vi "Project Save As.vi"(8 "error in (no error)":errorcluster, 9 "Rename Items[]":T1[](array[typedef]), 10 "Existing Project Path":path, 11 "New Project Path":path) -> (0 "error out":errorcluster)   [LabVIEW 2016, in "SLL Scripting.lvlib"]
uses:
  SLL Scripting.lvlib
  _Typedefs/Rename Item Cluster.ctl
  <vilib>/Utility/EditLVProj/Edit LVProj.lvlib
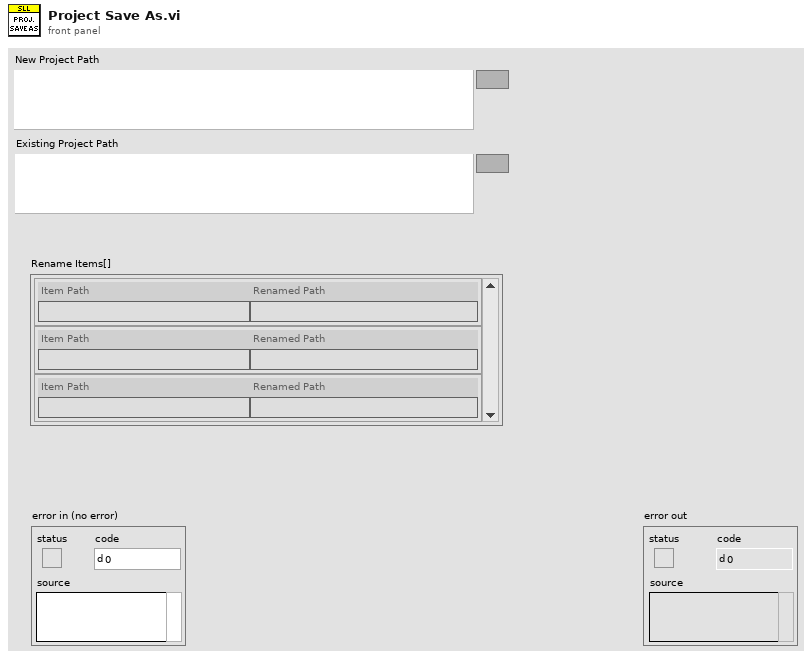
[diagram p1: front panel]
types:
  T1 = typedef "Rename Item Cluster.ctl" = cluster{"Item Path":string, "Renamed Path":string}
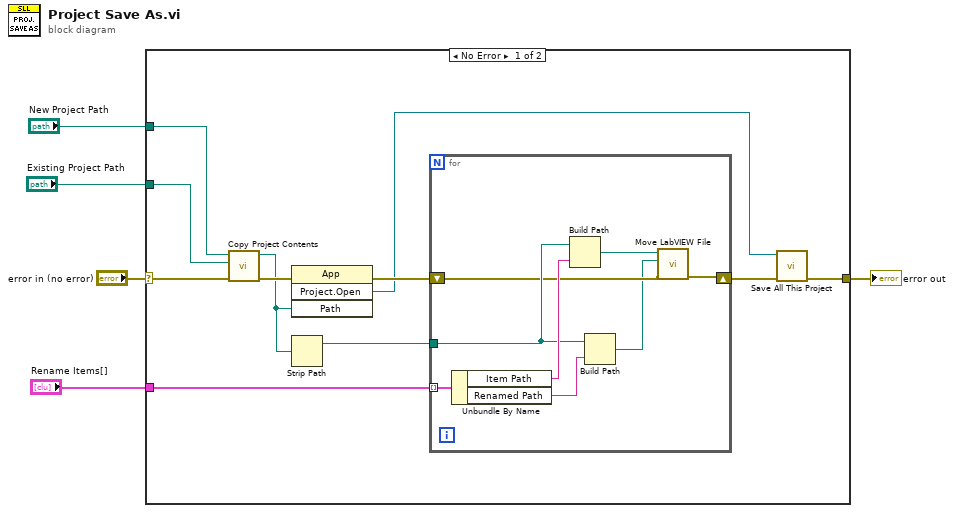
[diagram p0: block diagram]
diagram:
  n1 = case shown="No Error" "error in (no error)" {
    selector: "error in (no error)" -> [w16 w25]
    tunnel: [w7 w25] -> w4
    tunnel: "Existing Project Path" -> [w14 _]
    tunnel: "New Project Path" -> [w15 _]
    tunnel: "Rename Items[]" -> [w11 _]
    frame No Error {
      n2 = call "Copy Project Contents.vi"("error in (no error)"=w16, "Existing Project Path"=w14, "New Project Path"=w15) -> ("error out"=w13:errorcluster, "New Project Path Out"=w10:path)  [unwired: 7 in]
      n3 = invoke class="App" method="Project.Open"(error in=w13, "Path"=w10) -> (error out=w12:errorcluster, "Project:Open"=w6:refnum<vi>)  [unwired: 2 in, 2 out]
      n4 = Strip Path(path=w10) -> (stripped path=w9:path)  [unwired: 1 out]
      n5 = for {
        shift-right: [w17] -> w8
        shift-left: w12 -> [w20]
        tunnel: w11 -> [w24] mode=indexing
        tunnel: w9 -> [w22]
        n6 = Unbundle By Name(w24) -> ("Item Path"=w23:string, "Renamed Path"=w21:string)
        n7 = Build Path(base path=w22, name or relative path=w23) -> (appended path=w19:path)
        n8 = Build Path(base path=w22, name or relative path=w21) -> (appended path=w18:path)
        n9 = call "Move LabVIEW File.vi"("error in (no error)"=w20, "New Path"=w18, "Existing Path"=w19) -> ("error out"=w17:errorcluster)  [unwired: 8 in]
      }
      n10 = call <vilib>:"Save All This Project.vi"("error in (no error)"=w8, "Project in"=w6) -> ("error out"=w7:errorcluster)  [unwired: 8 in, 1 out]
    }
    frame Error {
    }
  }
  "error out" <- w4
